vi "AxisControl.vi"(0 "String in":string, 1 "AxisBounds":T5={"Min"={"Auto"=TRUE, "Value"=0.0}, "Max"={"Auto"=TRUE, "Value"=0.0}}, 3 "ticsAndGrids":T2={"tics"={"ticMin"=0.0, "ticStep"=0.0, "ticMax"=0.0, "minorDivsPerMajor"=2, "Mirror tics"=TRUE, "ticSpacing"=enum."Auto Tics"}, "Grids"={"Gridlines"=enum."Major grid", "Zeroaxis"=enum."No zero axis"}}, 5 "Axis":T7="x", 9 "ShowNumbers?":bool=TRUE, 11 "ShowLabel?":bool=TRUE, 12 "Axis Label":string, 13 "AxisSpan":dbl) -> (4 "String out":string)   [LabVIEW 2012]
uses:
  axisName.ctl
  minAndMax.ctl
  AutoManualNumber.ctl
  ticsAndGrids.ctl
  tics.ctl
  grids.ctl
  commandArray.ctl
panel:
  out "Commands":T1
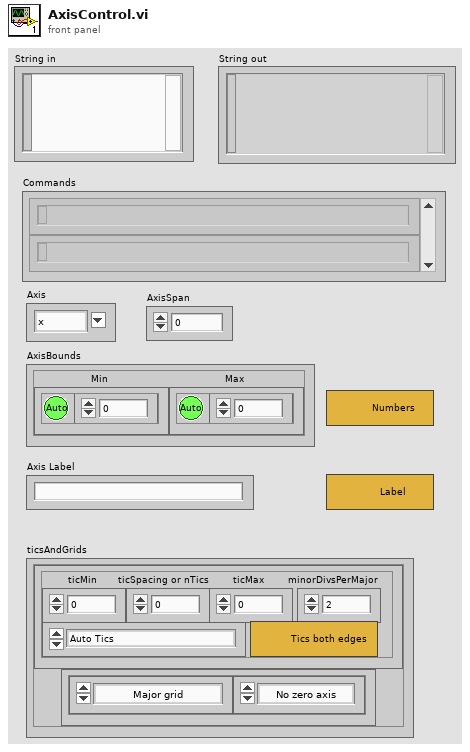
[diagram p1: front panel]
types:
  T1 = typedef "commandArray.ctl" = string[]
  T2 = typedef "ticsAndGrids.ctl" = cluster{"tics":T3, "Grids":T4}
  T3 = typedef "tics.ctl" = cluster{"ticMin":dbl, "ticStep":dbl, "ticMax":dbl, "minorDivsPerMajor":i32, "Mirror tics":bool, "ticSpacing":enum16{"Auto Tics", "Fixed spacing", "Fixed Minimum and Spacing", "Start, Spacing and Maximum", "Approx n Tics (rounded)"}}
  T4 = typedef "grids.ctl" = cluster{"Gridlines":enum16{"No grids", "Major grid", "Minor grid", "Major and Minor"}, "Zeroaxis":enum16{"No zero axis", "Show zero axis"}}
  T5 = typedef "minAndMax.ctl" = cluster{"Min":T6, "Max":T6}
  T6 = typedef "AutoManualNumber.ctl" = cluster{"Auto":bool, "Value":dbl}
  T7 = typedef "axisName.ctl" = string
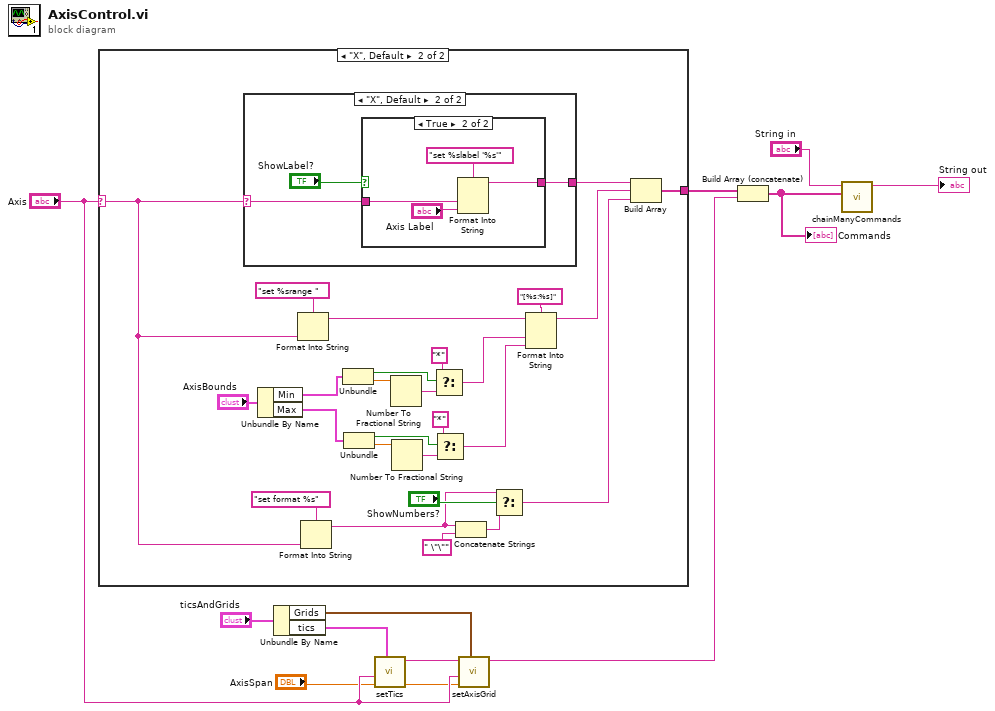
[diagram p0: block diagram]
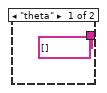
[diagram p2: hidden frame]
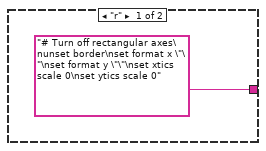
[diagram p3: hidden frame]
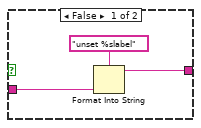
[diagram p4: hidden frame]
diagram:
  n1 = case shown="\"X\", Default" "Axis" {
    selector: "Axis" -> [_ w14]
    tunnel: [string[] [] w31] -> w8
    frame "theta" {
    }
    frame "X", Default {
      n2 = case shown="\"X\", Default" w14 {
        selector: w14 -> [_ w41]
        tunnel: ["# Turn off rectangular axes\nunset border\nset format x \"\"\nset format y \"\"\nset xtics scale 0\nset ytics scale 0" w42] -> w29
        frame "r" {
        }
        frame "X", Default {
          n3 = case shown="True" "ShowLabel?" {
            tunnel: w41 -> [w45 w48]
            tunnel: [w44 w47] -> w42
            frame False {
              n4 = Format Into String(format string="unset %slabel", w45) -> (resulting string=w44:string)  [unwired: 2 in, 1 out]
            }
            frame True {
              n5 = Format Into String(format string="set %slabel '%s'", w48, "Axis Label") -> (resulting string=w47:string)  [unwired: 2 in, 1 out]
            }
          }
        }
      }
      n6 = Unbundle By Name("AxisBounds") -> ("Min"=w16:T6, "Max"=w15:T6)
      n7 = Format Into String(format string="set %srange ", w14) -> (resulting string=w38:string)  [unwired: 2 in, 1 out]
      n8 = Format Into String(format string="set format %s", w14) -> (resulting string=w33:string)  [unwired: 2 in, 1 out]
      n9 = Unbundle(w16) -> ("Auto"=w24:bool, "Value"=w26:dbl)
      n10 = Unbundle(w15) -> ("Auto"=w22:bool, "Value"=w20:dbl)
      n11 = Number To Fractional String(number=w26) -> (F-format string=w27:string)  [unwired: 3 in]
      n12 = Number To Fractional String(number=w20) -> (F-format string=w19:string)  [unwired: 3 in]
      n13 = Select(t="*", s=w24, f=w27) -> (s? t:f=w23:string)
      n14 = Select(t="*", s=w22, f=w19) -> (s? t:f=w18:string)
      n15 = Concatenate Strings(w33, " \"\"" ("format string")) -> (w32:string)
      n16 = Select(t=w33, s="ShowNumbers?", f=w32) -> (s? t:f=w30:string)
      n17 = Format Into String(format string="[%s:%s]", initial string=w38, w23, w18) -> (resulting string=w37:string)  [unwired: 1 in, 1 out]
      n18 = Build Array(w29, w37, w30) -> (w31:string[])
    }
  }
  n19 = Unbundle By Name("ticsAndGrids") -> ("Grids"=w9:T4, "tics"=w10:T3)
  n20 = call "setTics.vi"("tics"=w10, "AxisSpan"="AxisSpan", "Axis"="Axis") -> ("polarGrid"=w5:dbl, "String out"=w11:string)  [unwired: 7 in]
  n21 = call "setAxisGrid.vi"("Grids"=w9, "polarGridAngle"=w5, "Axis"="Axis", "String in"=w11) -> ("String out"=w7:string)  [unwired: 7 in]
  n22 = Build Array (concatenate)(w8, w7) -> (w2:string[])
  "Commands" <- w2
  n23 = call "chainManyCommands.vi"("CommandArray"=w2, "String in in"="String in") -> ("String out"=→"String out":string)  [unwired: 9 in]
